vi "S2C_CMD_ManageCustTypes.vi"(8 "Error In":errorcluster, 10 "Default":string, 11 "Type":string) -> (0 "Error Out":errorcluster, 2 "Value_Int":string, 3 "Value_String":string)   [LabVIEW 2015]
doc: "Performs a lookup for the Int value associated with the input type default value, or the first Int value if no default is specified."
uses:
  S2C_CMD_Globals.vi
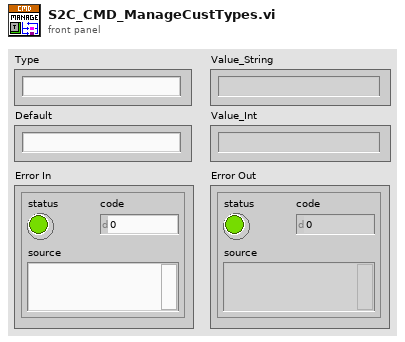
[diagram p1: front panel]
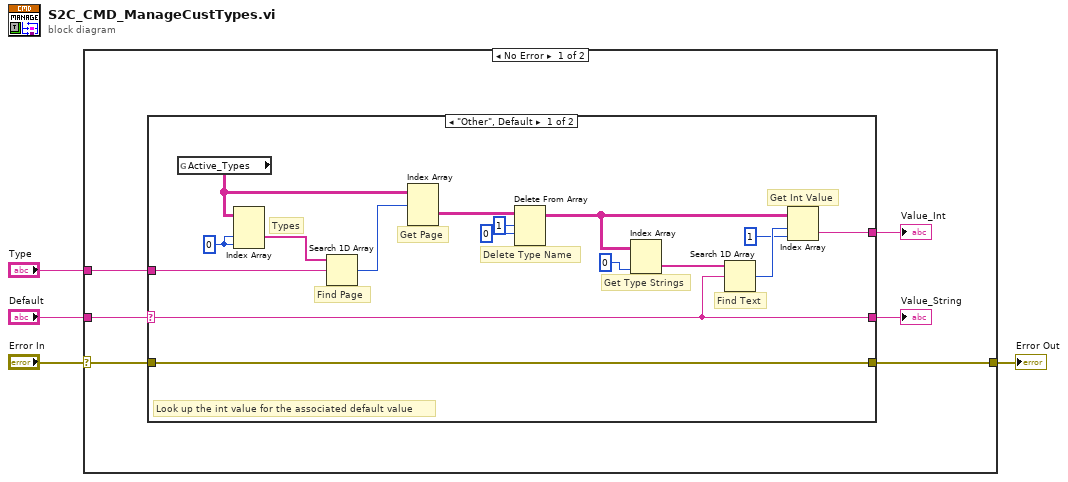
[diagram p0: block diagram]
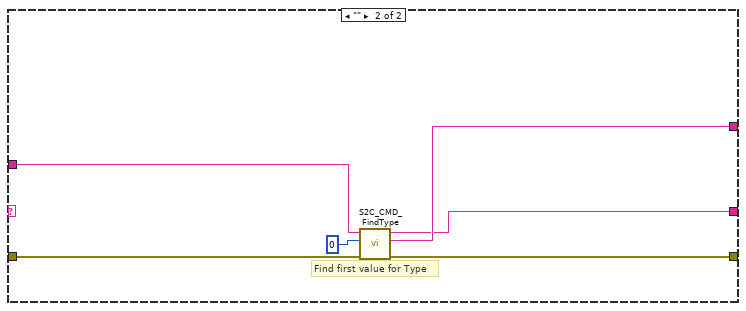
[diagram p2: hidden frame]
diagram:
  n1 = case shown="No Error" "Error In" {
    selector: "Error In" -> [w7 w33]
    tunnel: "Type" -> [w10 _]
    tunnel: [w6 w33] -> w2
    tunnel: "Default" -> [w8 _]
    frame No Error {
      n2 = case shown="\"Other\", Default" w8 {
        selector: w8 -> [w12 _]
        tunnel: w10 -> [w26 w27]
        tunnel: [w13 w29] -> w9
        tunnel: w7 -> [w11 w31]
        tunnel: [w11 w30] -> w6
        tunnel: [w12 w28] -> w5
        frame "Other", Default {
          w23 = 0 ("disabled index (row)")
          # "Look up the int value for the associated default value"
          # "Get Int Value"
          # "Find Text"
          # "Get Type Strings"
          # "Delete Type Name"
          # "Get Page"
          # "Find Page"
          # "Types"
          n3 = global read "S2C_CMD_Globals.vi" "Active_Types"() -> (w19:string[][][])
          n4 = Index Array(array=w19, index (dim 1)=w23, index (dim 2)=w23) -> (element=w22:string[])  [unwired: 1 in]
          n5 = Search 1D Array(1D array=w22, element=w26) -> (index of element=w20:i32)  [unwired: 1 in]
          n6 = Index Array(array=w19, index (dim 0)=w20) -> (element=w21:string[][])  [unwired: 2 in]
          n7 = Delete From Array(array=w21, length=1, index (row)=0) -> (array with subset deleted=w16:string[][])  [unwired: 1 in, 1 out]
          n8 = Index Array(array=w16, index (col)=0 ("disabled index (col)")) -> (element=w17:string[])  [unwired: 1 in]
          n9 = Search 1D Array(1D array=w17, element=w12) -> (index of element=w15:i32)  [unwired: 1 in]
          n10 = Index Array(array=w16, index (row)=w15, index (col)=1 ("disabled index (col)")) -> (element=w13:string)
        }
        frame "" {
          # "Find first value for Type"
          n11 = call "S2C_CMD_FindType.vi"("Error In"=w31, "Index"=0, "TypeString"=w27) -> ("Error Out"=w30:errorcluster, "Value_Int"=w29:string, "Value_Text"=w28:string)  [unwired: 4 in, 2 out]
        }
      }
      "Value_Int" <- w9
      "Value_String" <- w5
    }
    frame Error {
    }
  }
  "Error Out" <- w2
